vi "GetSortedSplitters.vi"(8 "error in (no error)":errorcluster, 10 "Height":u32, 11 "Splitters[]":refnum<vi>[](array[refnum])) -> (0 "error out":errorcluster, 1 "2 Vert and 2 Horiz Splitters?":bool, 2 "Splitters":T1, 3 "Same size Splitters?":bool, 4 "Vertical on Top?":bool, 5 "Number of Splitters":i32)   [LabVIEW 2022 SP3, in "PentaPanesLibrary.lvlib" / "PentaPanes.lvclass"]
uses:
  PentaPanes.lvclass
  SplittersCluster.ctl
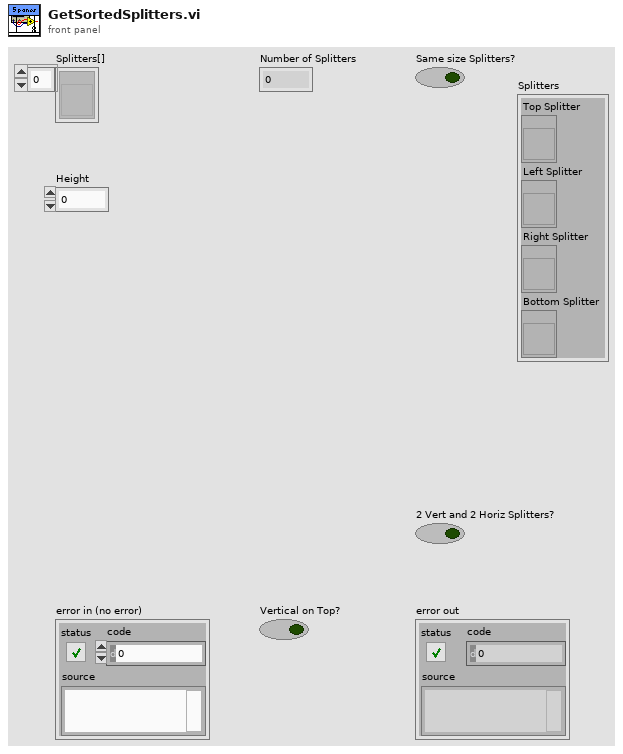
[diagram p1: front panel]
types:
  T1 = typedef "PentaPanesLibrary.lvlib/PentaPanes.lvclass/SplittersCluster.ctl" = cluster{"Top Splitter":refnum<vi>, "Left Splitter":refnum<vi>, "Right Splitter":refnum<vi>, "Bottom Splitter":refnum<vi>}
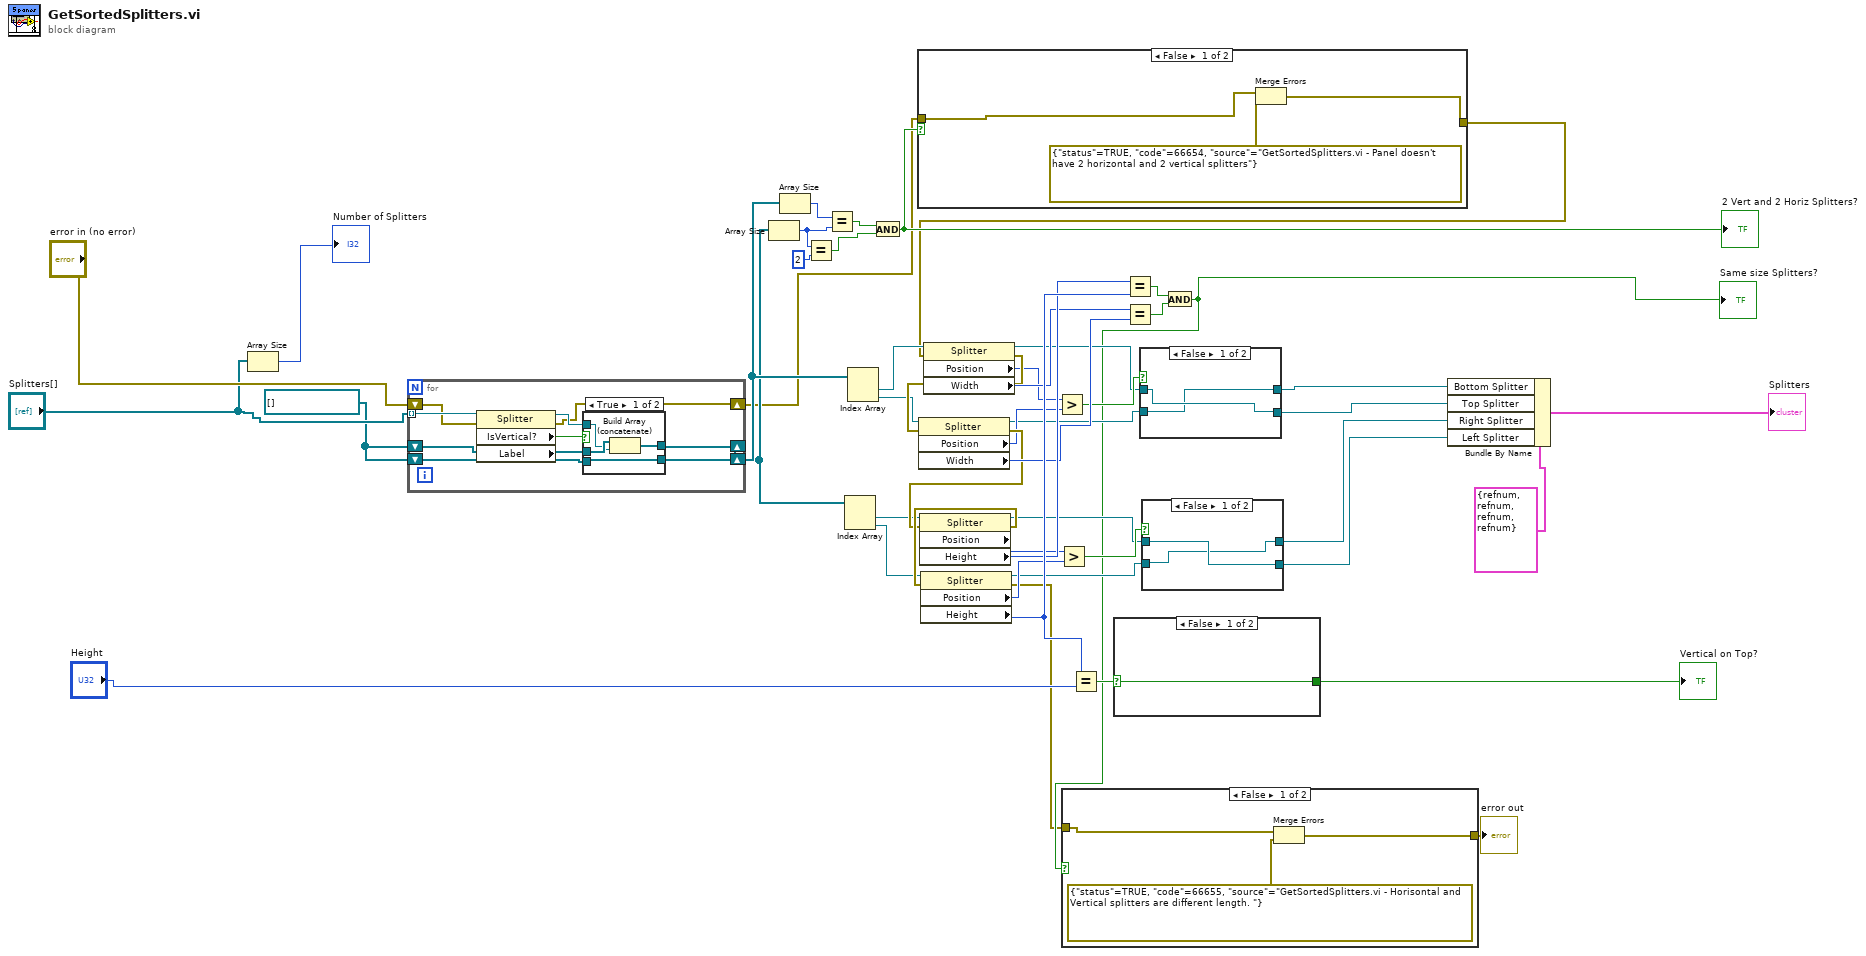
[diagram p0: block diagram]
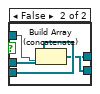
[diagram p7: hidden frame]
diagram:
  w34 = refnum<vi>[] [] ("Splitters[]")
  n1 = Array Size(array="Splitters[]") -> (size(s)=→"Number of Splitters":i32)
  n2 = for {
    tunnel: "Splitters[]" -> [w58] mode=indexing
    shift-right: [w52] -> w28
    shift-left: w34 -> [w53]
    shift-right: [w54] -> w9
    shift-left: w34 -> [w56]
    shift-right: [w50] -> w6
    shift-left: "error in (no error)" -> [w51]
    n3 = property class="Splitter" props=["IsVertical?", "Label"](reference=w58, error in=w51) -> (reference out=w55:refnum<vi>, error out=w50:errorcluster, "IsVertical?"=w57:bool)  [unwired: 1 out]
    n4 = case shown="True" w57 {
      tunnel: w56 -> [w62 w63]
      tunnel: w55 -> [w61 w66]
      tunnel: [w60 w63] -> w54
      tunnel: w53 -> [w59 w65]
      tunnel: [w59 w64] -> w52
      frame True {
        n5 = Build Array (concatenate)(w62, w61) -> (w60:refnum<vi>[])
      }
      frame False {
        n6 = Build Array (concatenate)(w65, w66) -> (w64:refnum<vi>[])
      }
    }
  }
  n7 = Array Size(array=w9) -> (size(s)=w32:i32)
  n8 = Array Size(array=w28) -> (size(s)=w33:i32)
  n9 = Equal?(x=w32, y=2) -> (x = y?=w29:bool)
  n10 = Equal?(x=w33, y=w32) -> (x = y?=w30:bool)
  n11 = Index Array(array=w9) -> (element #1=w13:refnum<vi>, element #2=w12:refnum<vi>)  [unwired: 2 in]
  n12 = Index Array(array=w28) -> (element #1=w27:refnum<vi>, element #2=w26:refnum<vi>)  [unwired: 2 in]
  n13 = And(x=w30, y=w29) -> (x .and. y?=w8:bool)
  "2 Vert and 2 Horiz Splitters?" <- w8
  n14 = case shown="False" w8 {
    tunnel: w6 -> [w69 w70]
    tunnel: [w67 w70] -> w5
    frame False {
      n15 = Merge Errors(w69, errorcluster {"status"=TRUE, "code"=66654, "source"="GetSortedSplitters.vi - Panel doesn't have 2 horizontal and 2 vertical splitters"} ("error out")) -> (w67:errorcluster)
    }
    frame True {
    }
  }
  n16 = property class="Splitter"(reference=w27, error in=w5) -> (reference out=w22:refnum<vi>, error out=w38:errorcluster, "Position"=w25:i32, "Width"=w44:u32)
  n17 = property class="Splitter"(reference=w26, error in=w38) -> (reference out=w21:refnum<vi>, error out=w39:errorcluster, "Position"=w24:i32, "Width"=w45:u32)
  n18 = property class="Splitter"(reference=w13, error in=w39) -> (reference out=w17:refnum<vi>, error out=w40:errorcluster, "Position"=w20:i32, "Height"=w46:u32)
  n19 = property class="Splitter"(reference=w12, error in=w40) -> (reference out=w16:refnum<vi>, error out=w4:errorcluster, "Position"=w19:i32, "Height"=w47:u32)
  n20 = Greater?(x=w25, y=w24) -> (0:w23:bool)
  n21 = Greater?(x=w20, y=w19) -> (0:w18:bool)
  n22 = Equal?(x=w47, y="Height") -> (x = y?=w41:bool)
  n23 = case shown="False" w41 {
    selector: w41 -> [w71 w72]
    tunnel: [w71 w72] -> w43
    frame False {
    }
    frame True {
    }
  }
  "Vertical on Top?" <- w43
  n24 = Equal?(x=w46, y=w47) -> (x = y?=w48:bool)
  n25 = Equal?(x=w44, y=w45) -> (x = y?=w49:bool)
  n26 = case shown="False" w23 {
    tunnel: w22 -> [w74 w76]
    tunnel: w21 -> [w73 w75]
    tunnel: [w73 w76] -> w10
    tunnel: [w74 w75] -> w11
    frame False {
    }
    frame True {
    }
  }
  n27 = case shown="False" w18 {
    tunnel: w17 -> [w78 w80]
    tunnel: w16 -> [w77 w79]
    tunnel: [w77 w80] -> w15
    tunnel: [w78 w79] -> w14
    frame False {
    }
    frame True {
    }
  }
  n28 = And(x=w48, y=w49) -> (x .and. y?=w7:bool)
  "Same size Splitters?" <- w7
  n29 = case shown="False" w7 {
    tunnel: w4 -> [w83 w84]
    tunnel: [w81 w84] -> w3
    frame False {
      n30 = Merge Errors(w83, errorcluster {"status"=TRUE, "code"=66655, "source"="GetSortedSplitters.vi - Horisontal and Vertical splitters are different length. "} ("error out")) -> (w81:errorcluster)
    }
    frame True {
    }
  }
  "error out" <- w3
  n31 = Bundle By Name(cluster=T1 {"Top Splitter"=refnum, "Left Splitter"=refnum, "Right Splitter"=refnum, "Bottom Splitter"=refnum} ("Splitters"), "Bottom Splitter"=w10, "Top Splitter"=w11, "Right Splitter"=w15, "Left Splitter"=w14) -> (→"Splitters":T1)
